vi "Motion Profile Generater.vi"() -> ()   [LabVIEW 2015]
panel:
  out "XY Graph":cluster{dbl[], dbl[]}[](graph)
  in  "Motion Profile Control Frame Rate":dbl
  in  "Max Jerk (rotations/sec^3)":dbl
  in  "Max Acceleration (rotations/sec^2)":dbl
  in  "Rotations to Travel":dbl
  in  "Max Speed (rotations/sec)":dbl
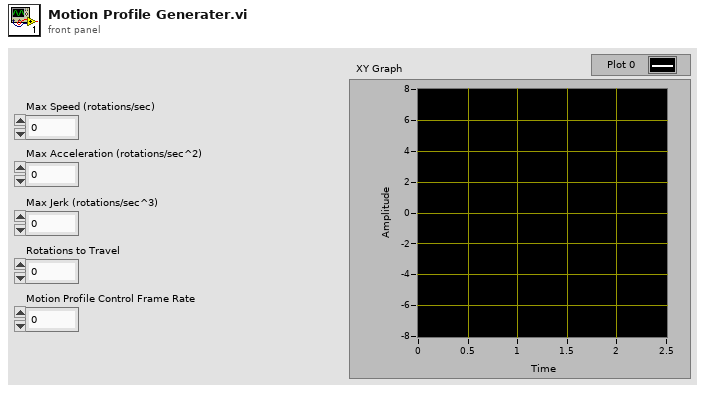
[diagram p1: front panel]
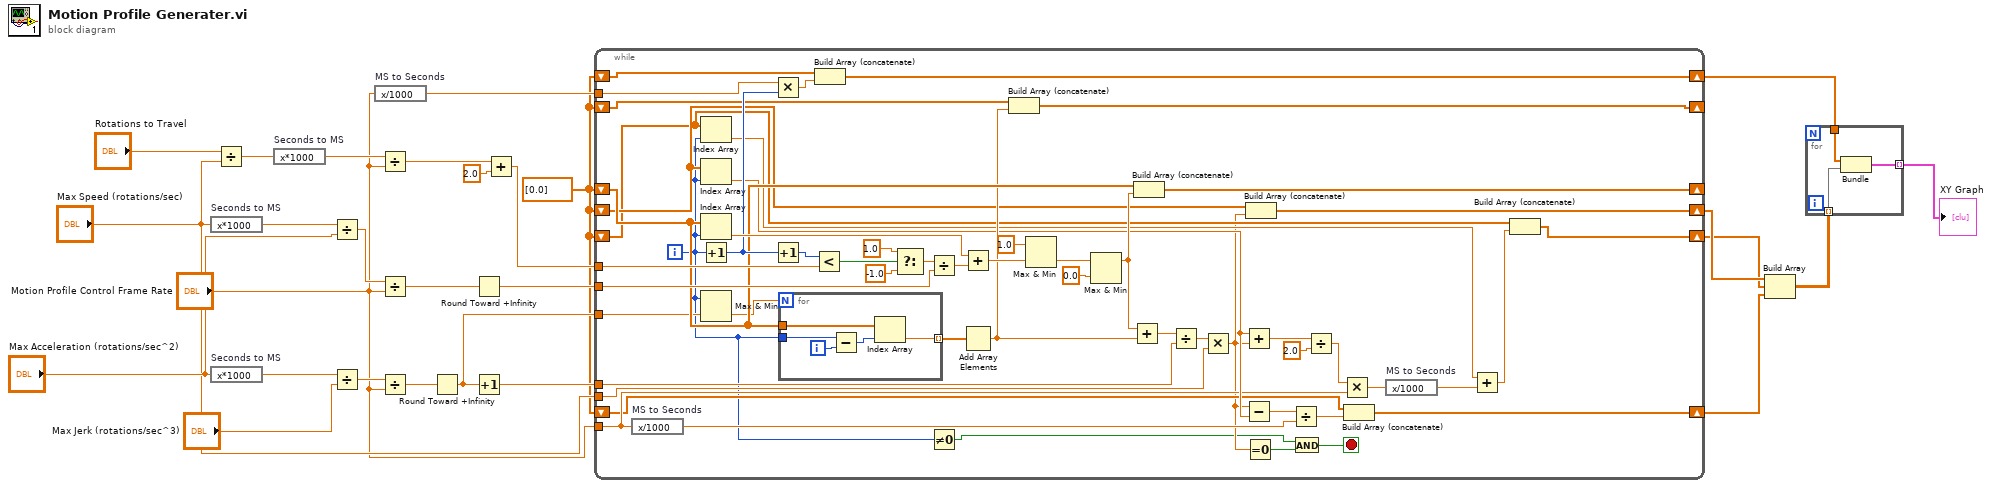
[diagram p0: block diagram]
diagram:
  w7 = dbl[] [0.0]
  n1 = expression code="x*1000" "Seconds to MS"("Max Speed (rotations/sec)") -> (w23:dbl)
  n2 = expression code="x*1000" "Seconds to MS"("Max Acceleration (rotations/sec^2)") -> (w24:dbl)
  n3 = Divide(x="Rotations to Travel", y="Max Speed (rotations/sec)") -> (x/y=w21:dbl)
  n4 = expression code="x*1000" "Seconds to MS"(w21) -> (w20:dbl)
  n5 = Divide(x=w23, y="Max Acceleration (rotations/sec^2)") -> (x/y=w16:dbl)
  n6 = Divide(x=w24, y="Max Jerk (rotations/sec^3)") -> (x/y=w13:dbl)
  n7 = expression code="x/1000" "MS to Seconds"("Motion Profile Control Frame Rate") -> (w26:dbl)
  n8 = Divide(x=w20, y="Motion Profile Control Frame Rate") -> (x/y=w19:dbl)
  n9 = Divide(x=w16, y="Motion Profile Control Frame Rate") -> (x/y=w15:dbl)
  n10 = Divide(x=w13, y="Motion Profile Control Frame Rate") -> (x/y=w12:dbl)
  n11 = Round Toward +Infinity(x=w12) -> (ceil(x): smallest int >= x=w11:dbl)
  n12 = Round Toward +Infinity(x=w15) -> (ceil(x): smallest int >= x=w14:dbl)
  n13 = Increment(x=w11) -> (x+1=w10:dbl)
  n14 = Add(x=w19, y=2.0) -> (x+y=w17:dbl)
  n15 = while {
    shift-right: [w80] -> w2
    shift-left: w7 -> [w81]
    tunnel: w26 -> [w79]
    tunnel: w17 -> [w77]
    shift-right: [w63] -> _
    shift-left: w7 -> [w62]
    tunnel: w14 -> [w69]
    tunnel: w11 -> [w60]
    shift-right: [w57] -> _
    shift-left: w7 -> [w58]
    tunnel: w10 -> [w53]
    tunnel: "Max Speed (rotations/sec)" -> [w51]
    shift-right: [w50] -> w6
    shift-left: w7 -> [w48]
    shift-right: [w49] -> w5
    shift-left: w7 -> [w42]
    tunnel: "Motion Profile Control Frame Rate" -> [w36]
    shift-right: [w34] -> w4
    shift-left: w7 -> [w33]
    i -> [w32]
    stop <- w28 stop-if-true
    n16 = expression code="x/1000" "MS to Seconds"(w36) -> (w37:dbl)
    n17 = Index Array(array=w42, index=w32) -> (element=w41:dbl)
    n18 = Index Array(array=w48, index=w32) -> (element=w39:dbl)
    n19 = Index Array(array=w62, index=w32) -> (element=w67:dbl)
    n20 = Increment(x=w32) -> (x+1=w65:i32)
    n21 = Max & Min(x=w32, y=w60) -> (min(x,y)=w59:dbl)  [unwired: 1 out]
    n22 = Multiply(x=w79, y=w65) -> (x*y=w78:dbl)
    n23 = Increment(x=w65) -> (x+1=w66:i32)
    n24 = for {
      N: w59 -> [_]
      tunnel: w32 -> [w85]
      tunnel: w62 -> [w83]
      tunnel: [w82] -> w61 mode=indexing
      i -> [w86]
      n25 = Subtract(x=w85, y=w86) -> (x-y=w84:i32)
      n26 = Index Array(array=w83, index=w84) -> (element=w82:dbl)
    }
    n27 = Less?(x=w66, y=w77) -> (x < y?=w73:bool)
    n28 = Build Array (concatenate)(w81, w78) -> (w80:dbl[])
    n29 = Select(t=1.0, s=w73, f=-1.0) -> (s? t:f=w70:dbl)
    n30 = Divide(x=w70, y=w69) -> (x/y=w68:dbl)
    n31 = Not Equal To 0?(x=w32) -> (x != 0?=w29:bool)
    n32 = Add(x=w67, y=w68) -> (x+y=w64:dbl)
    n33 = Add Array Elements(numeric array=w61) -> (sum=w56:dbl)
    n34 = Build Array (concatenate)(w58, w56) -> (w57:dbl[])
    n35 = Max & Min(x=1.0, y=w64) -> (min(x,y)=w75:dbl)  [unwired: 1 out]
    n36 = Max & Min(x=w75, y=0.0) -> (max(x,y)=w55:dbl)  [unwired: 1 out]
    n37 = Add(x=w55, y=w56) -> (x+y=w54:dbl)
    n38 = Build Array (concatenate)(w62, w55) -> (w63:dbl[])
    n39 = Divide(x=w54, y=w53) -> (x/y=w52:dbl)
    n40 = Multiply(x=w52, y=w51) -> (x*y=w31:dbl)
    n41 = Add(x=w39, y=w31) -> (x+y=w47:dbl)
    n42 = Subtract(x=w31, y=w39) -> (x-y=w38:dbl)
    n43 = Equal To 0?(x=w31) -> (x = 0?=w30:bool)
    n44 = Build Array (concatenate)(w48, w31) -> (w50:dbl[])
    n45 = Divide(x=w38, y=w37) -> (x/y=w35:dbl)
    n46 = And(x=w29, y=w30) -> (x .and. y?=w28:bool)
    n47 = Divide(x=w47, y=2.0) -> (x/y=w45:dbl)
    n48 = Multiply(x=w45, y=w36) -> (x*y=w44:dbl)
    n49 = Build Array (concatenate)(w33, w35) -> (w34:dbl[])
    n50 = expression code="x/1000" "MS to Seconds"(w44) -> (w43:dbl)
    n51 = Add(x=w41, y=w43) -> (x+y=w40:dbl)
    n52 = Build Array (concatenate)(w42, w40) -> (w49:dbl[])
  }
  n53 = Build Array(w6, w5, w4) -> (w3:dbl[][])
  n54 = for {
    tunnel: w3 -> [w89] mode=indexing
    tunnel: w2 -> [w88]
    tunnel: [w87] -> w1 mode=indexing
    n55 = Bundle(w88, w89) -> (w87:cluster{dbl[], dbl[]})  [unwired: 1 in]
  }
  "XY Graph" <- w1
